vi "parse message read.vi"(9 "# of messages":i32=6, 10 "Raw Data In":u8[](array[numeric])=array[481600 elements]) -> (2 "Messages out":T1[](array[typedef]) {"AckBytes [8]" format="%.0x"; "Data [8]" format="%.0x"; "ArbIDOrHeader" format="%.0x"; "DescriptionID" format="%.0x"; "NetworkID" format="%.0x"})   [LabVIEW 2009]
uses:
  ctl spymessage.ctl
panel:
  out "subarray":u8[][](array[numeric])
  out "Array":u8[](array[numeric])
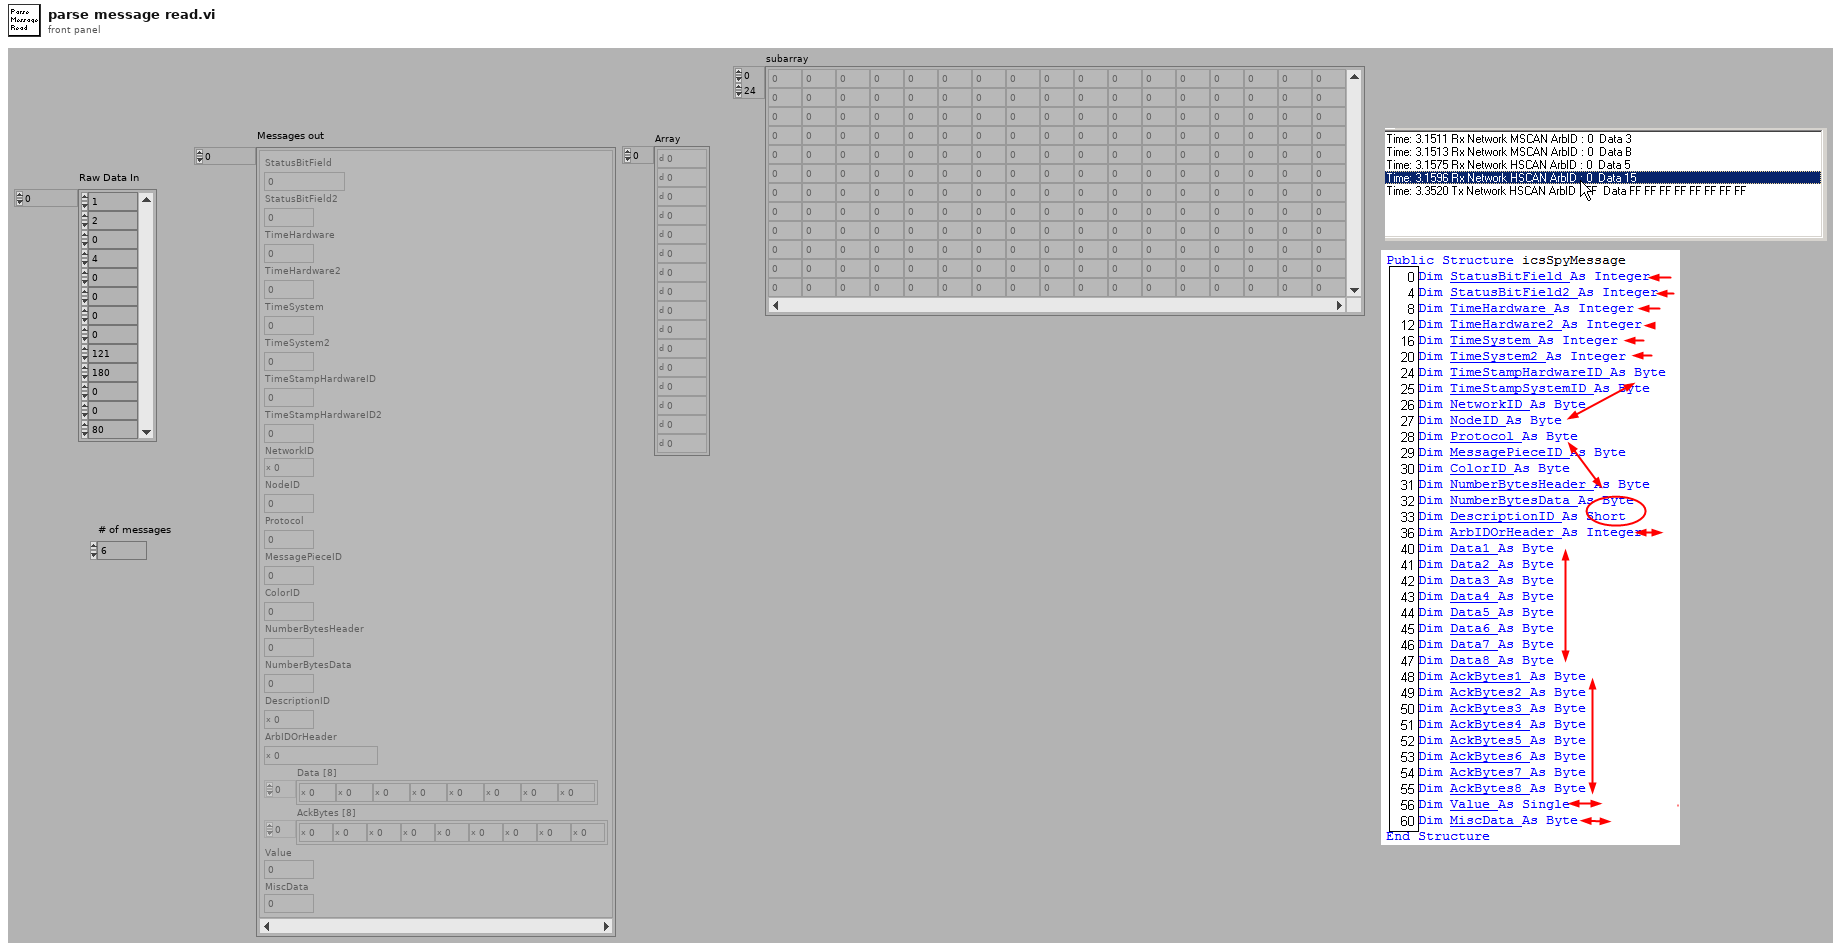
[diagram p1: front panel]
types:
  T1 = typedef "ctl spymessage.ctl" = cluster{"StatusBitField":u32, "StatusBitField2":u32, "TimeHardware":u32, "TimeHardware2":u32, "TimeSystem":u32, "TimeSystem2":u32, "TimeStampHardwareID":u8, "TimeStampHardwareID2":u8, "NetworkID":u8, "NodeID":u8, "Protocol":u8, "MessagePieceID":u8, "ColorID":u8, "NumberBytesHeader":u8, "NumberBytesData":u8, "DescriptionID":u16, "ArbIDOrHeader":u32, "Data [8]":u8[], "AckBytes [8]":u8[], "Value":sgl, "MiscData":u8}
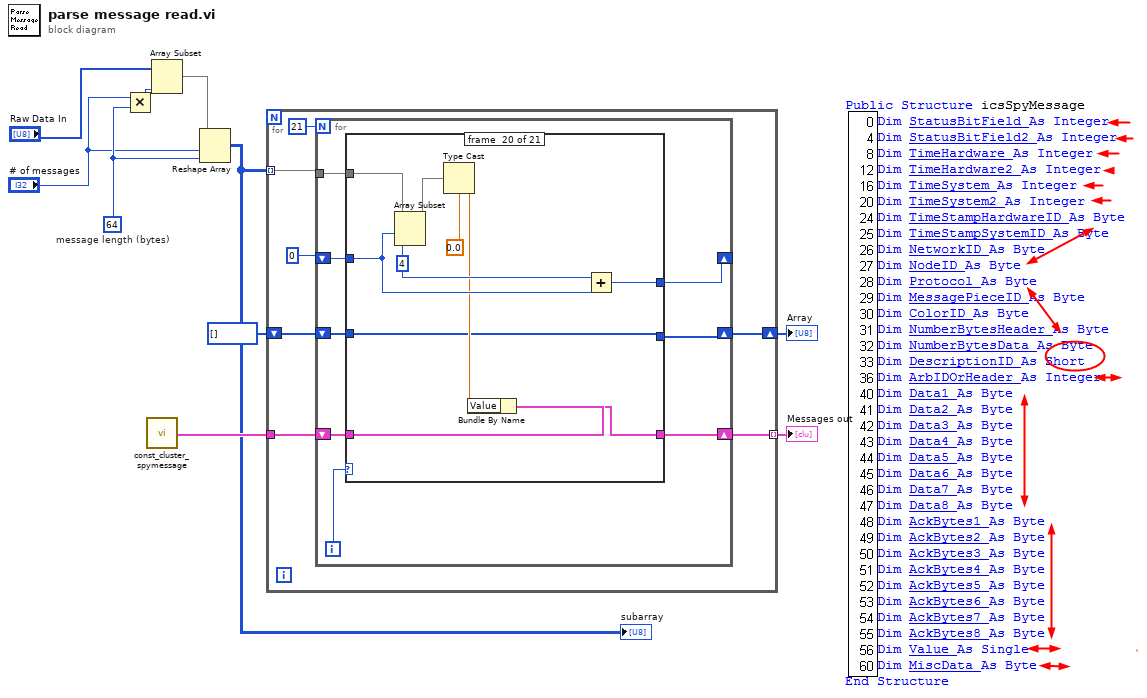
[diagram p0: block diagram]
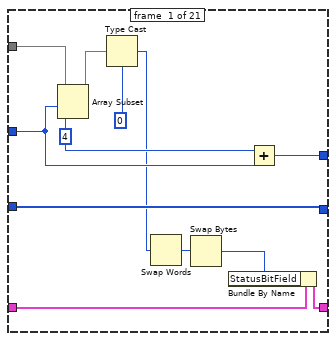
[diagram p2: hidden frame]
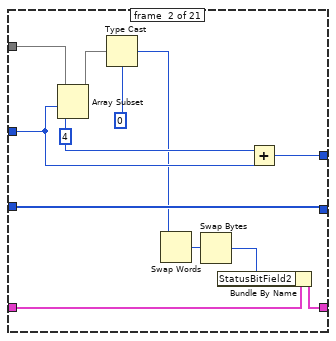
[diagram p3: hidden frame]
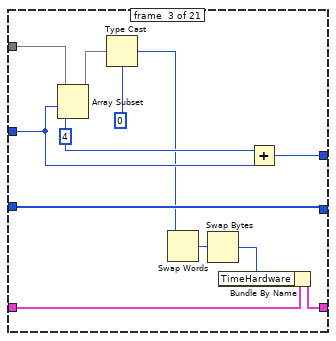
[diagram p4: hidden frame]
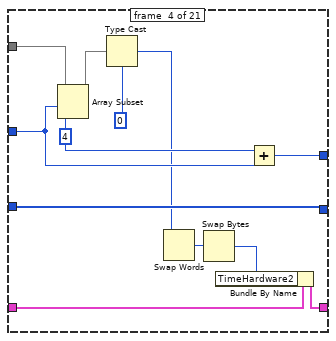
[diagram p5: hidden frame]
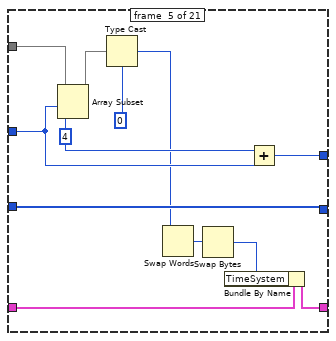
[diagram p6: hidden frame]
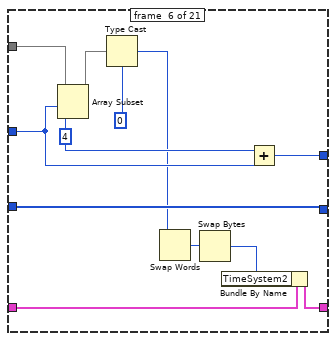
[diagram p7: hidden frame]
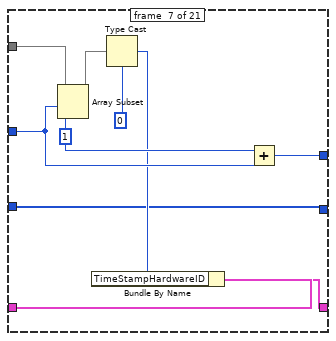
[diagram p8: hidden frame]
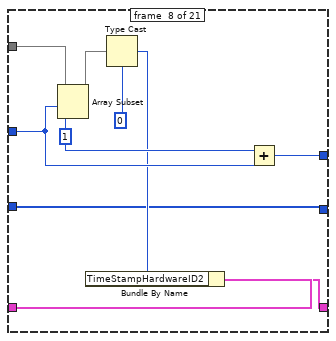
[diagram p9: hidden frame]
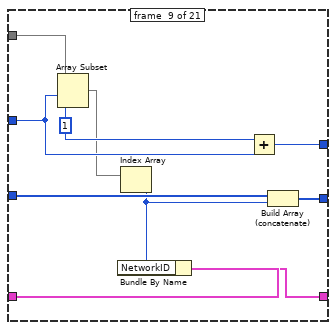
[diagram p10: hidden frame]
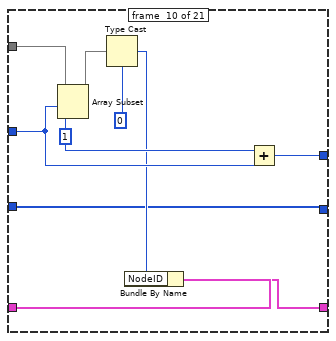
[diagram p11: hidden frame]
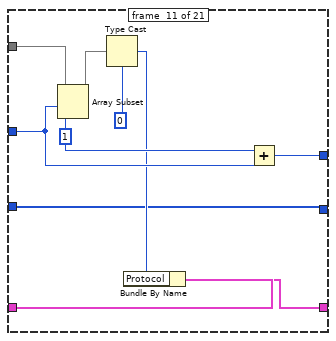
[diagram p12: hidden frame]
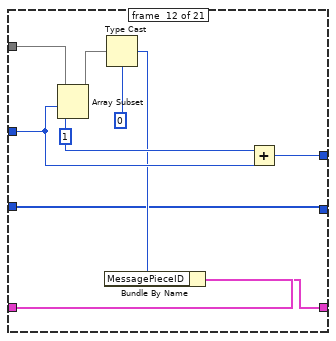
[diagram p13: hidden frame]
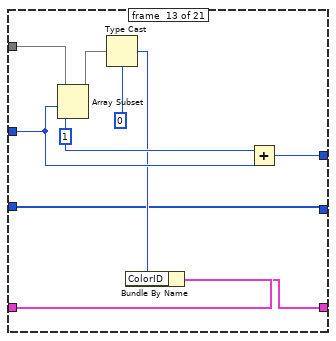
[diagram p14: hidden frame]
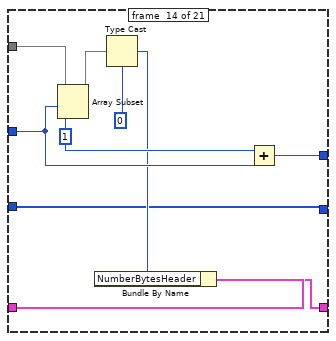
[diagram p15: hidden frame]
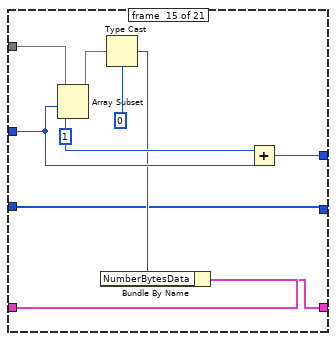
[diagram p16: hidden frame]
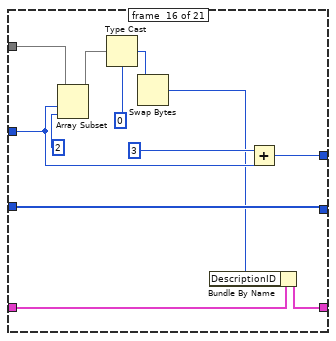
[diagram p17: hidden frame]
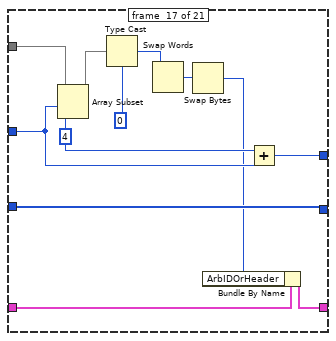
[diagram p18: hidden frame]
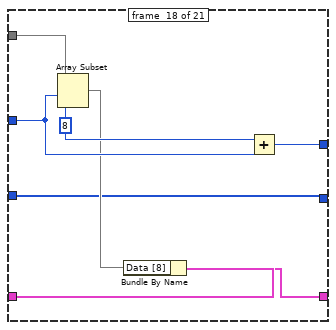
[diagram p19: hidden frame]
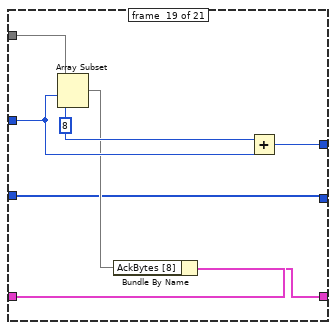
[diagram p20: hidden frame]
diagram:
  w5 = 64  # message length (bytes)
  n1 = Multiply(x="# of messages", y=w5) -> (x*y=w4:i32)
  n2 = call "const_cluster_spymessage.vi"() -> ("SpyMessage{}"=w10:T1)
  n3 = Array Subset(array="Raw Data In", length=w4) -> (w3:u8[])  [unwired: 1 in]
  n4 = Reshape Array(w3, "# of messages", w5) -> (w1:u8[][])
  "subarray" <- w1
  n5 = for {
    tunnel: w1 -> [w17] mode=indexing
    tunnel: w10 -> [w16]
    tunnel: [w13] -> w9 mode=indexing
    shift-right: [w11] -> w7
    shift-left: u8[] [] -> [w12]
    n6 = for {
      N: 21 -> [_]
      tunnel: w17 -> [w25]
      shift-right: [w20] -> _
      shift-left: 0 -> [w21]
      shift-right: [w22] -> w13
      shift-left: w16 -> [w23]
      shift-right: [w18] -> w11
      shift-left: w12 -> [w19]
      i -> [w24]
      n7 = case shown="8" w24 {
        tunnel: w25 -> [w35 w47 w59 w71 w83 w95 w105 w115 w125 w135 w145 w155 w165 w175 w185 w197 w209 w217 w225 w235 w246]
        tunnel: w23 -> [w37 w49 w61 w73 w85 w97 w107 w117 w127 w137 w147 w157 w167 w177 w187 w199 w211 w219 w227 w237 w248]
        tunnel: [w36 w48 w60 w72 w84 w96 w106 w116 w126 w136 w146 w156 w166 w176 w186 w198 w210 w218 w226 w236 w247] -> w22
        tunnel: w21 -> [w34 w46 w58 w70 w82 w94 w104 w114 w124 w134 w144 w154 w164 w174 w184 w196 w208 w216 w224 w234 w245]
        tunnel: [w32 w44 w56 w68 w80 w92 w102 w112 w122 w132 w142 w152 w162 w172 w182 w195 w206 w214 w222 w232 w243] -> w20
        tunnel: w19 -> [w29 w41 w53 w65 w77 w89 w98 w108 w121 w128 w138 w148 w158 w168 w178 w190 w203 w212 w220 w228 w238]
        tunnel: [w29 w41 w53 w65 w77 w89 w98 w108 w120 w128 w138 w148 w158 w168 w178 w190 w203 w212 w220 w228 w238] -> w18
        frame #0 {
          w33 = 4 ("length")
          n8 = Array Subset(array=w35, index=w34, length=w33) -> (w31:u8[])
          n9 = Type Cast(type=u32 0 ("length"), x=w31) -> (*(type *) &x=w27:u32)
          n10 = Swap Words(1:w27) -> (0:w28:u32)
          n11 = Swap Bytes(anything=w28) -> (byte swapped=w26:u32)
          n12 = Bundle By Name(cluster=w37, "StatusBitField"=w26) -> (w36:T1)
          n13 = Add(x=w33, y=w34) -> (x+y=w32:i32)
        }
        frame #1 {
          w45 = 4 ("length")
          n14 = Array Subset(array=w47, index=w46, length=w45) -> (w43:u8[])
          n15 = Type Cast(type=u32 0 ("length"), x=w43) -> (*(type *) &x=w39:u32)
          n16 = Swap Words(1:w39) -> (0:w40:u32)
          n17 = Swap Bytes(anything=w40) -> (byte swapped=w38:u32)
          n18 = Bundle By Name(cluster=w49, "StatusBitField2"=w38) -> (w48:T1)
          n19 = Add(x=w45, y=w46) -> (x+y=w44:i32)
        }
        frame #2 {
          w57 = 4 ("length")
          n20 = Array Subset(array=w59, index=w58, length=w57) -> (w55:u8[])
          n21 = Type Cast(type=u32 0 ("length"), x=w55) -> (*(type *) &x=w51:u32)
          n22 = Swap Words(1:w51) -> (0:w52:u32)
          n23 = Swap Bytes(anything=w52) -> (byte swapped=w50:u32)
          n24 = Bundle By Name(cluster=w61, "TimeHardware"=w50) -> (w60:T1)
          n25 = Add(x=w57, y=w58) -> (x+y=w56:i32)
        }
        frame #3 {
          w69 = 4 ("length")
          n26 = Array Subset(array=w71, index=w70, length=w69) -> (w67:u8[])
          n27 = Type Cast(type=0 ("length"), x=w67) -> (*(type *) &x=w63:i32)
          n28 = Swap Words(1:w63) -> (0:w64:i32)
          n29 = Swap Bytes(anything=w64) -> (byte swapped=w62:i32)
          n30 = Bundle By Name(cluster=w73, "TimeHardware2"=w62) -> (w72:T1)
          n31 = Add(x=w69, y=w70) -> (x+y=w68:i32)
        }
        frame #4 {
          w81 = 4 ("length")
          n32 = Array Subset(array=w83, index=w82, length=w81) -> (w79:u8[])
          n33 = Type Cast(type=0 ("length"), x=w79) -> (*(type *) &x=w75:i32)
          n34 = Swap Words(1:w75) -> (0:w76:i32)
          n35 = Swap Bytes(anything=w76) -> (byte swapped=w74:i32)
          n36 = Bundle By Name(cluster=w85, "TimeSystem"=w74) -> (w84:T1)
          n37 = Add(x=w81, y=w82) -> (x+y=w80:i32)
        }
        frame #5 {
          w93 = 4 ("length")
          n38 = Array Subset(array=w95, index=w94, length=w93) -> (w91:u8[])
          n39 = Type Cast(type=0 ("length"), x=w91) -> (*(type *) &x=w87:i32)
          n40 = Swap Words(1:w87) -> (0:w88:i32)
          n41 = Swap Bytes(anything=w88) -> (byte swapped=w86:i32)
          n42 = Bundle By Name(cluster=w97, "TimeSystem2"=w86) -> (w96:T1)
          n43 = Add(x=w93, y=w94) -> (x+y=w92:i32)
        }
        frame #6 {
          w103 = 1 ("length")
          n44 = Array Subset(array=w105, index=w104, length=w103) -> (w101:u8[])
          n45 = Type Cast(type=u8 0 ("length"), x=w101) -> (*(type *) &x=w99:u8)
          n46 = Bundle By Name(cluster=w107, "TimeStampHardwareID"=w99) -> (w106:T1)
          n47 = Add(x=w103, y=w104) -> (x+y=w102:i32)
        }
        frame #7 {
          w113 = 1 ("length")
          n48 = Array Subset(array=w115, index=w114, length=w113) -> (w111:u8[])
          n49 = Type Cast(type=u8 0 ("length"), x=w111) -> (*(type *) &x=w109:u8)
          n50 = Bundle By Name(cluster=w117, "TimeStampHardwareID2"=w109) -> (w116:T1)
          n51 = Add(x=w113, y=w114) -> (x+y=w112:i32)
        }
        frame #8 {
          w123 = 1 ("length")
          n52 = Array Subset(array=w125, index=w124, length=w123) -> (w119:u8[])
          n53 = Index Array(array=w119) -> (element=w118:u8)  [unwired: 1 in]
          n54 = Bundle By Name(cluster=w127, "NetworkID"=w118) -> (w126:T1)
          n55 = Add(x=w123, y=w124) -> (x+y=w122:i32)
          n56 = Build Array (concatenate)(w121, w118) -> (w120:u8[])
        }
        frame #9 {
          w133 = 1 ("length")
          n57 = Array Subset(array=w135, index=w134, length=w133) -> (w131:u8[])
          n58 = Type Cast(type=u8 0 ("length"), x=w131) -> (*(type *) &x=w129:u8)
          n59 = Bundle By Name(cluster=w137, "NodeID"=w129) -> (w136:T1)
          n60 = Add(x=w133, y=w134) -> (x+y=w132:i32)
        }
        frame #10 {
          w143 = 1 ("length")
          n61 = Array Subset(array=w145, index=w144, length=w143) -> (w141:u8[])
          n62 = Type Cast(type=u8 0 ("length"), x=w141) -> (*(type *) &x=w139:u8)
          n63 = Bundle By Name(cluster=w147, "Protocol"=w139) -> (w146:T1)
          n64 = Add(x=w143, y=w144) -> (x+y=w142:i32)
        }
        frame #11 {
          w153 = 1 ("length")
          n65 = Array Subset(array=w155, index=w154, length=w153) -> (w151:u8[])
          n66 = Type Cast(type=u8 0 ("length"), x=w151) -> (*(type *) &x=w149:u8)
          n67 = Bundle By Name(cluster=w157, "MessagePieceID"=w149) -> (w156:T1)
          n68 = Add(x=w153, y=w154) -> (x+y=w152:i32)
        }
        frame #12 {
          w163 = 1 ("length")
          n69 = Array Subset(array=w165, index=w164, length=w163) -> (w161:u8[])
          n70 = Type Cast(type=u8 0 ("length"), x=w161) -> (*(type *) &x=w159:u8)
          n71 = Bundle By Name(cluster=w167, "ColorID"=w159) -> (w166:T1)
          n72 = Add(x=w163, y=w164) -> (x+y=w162:i32)
        }
        frame #13 {
          w173 = 1 ("length")
          n73 = Array Subset(array=w175, index=w174, length=w173) -> (w171:u8[])
          n74 = Type Cast(type=u8 0 ("length"), x=w171) -> (*(type *) &x=w169:u8)
          n75 = Bundle By Name(cluster=w177, "NumberBytesHeader"=w169) -> (w176:T1)
          n76 = Add(x=w173, y=w174) -> (x+y=w172:i32)
        }
        frame #14 {
          w183 = 1 ("length")
          n77 = Array Subset(array=w185, index=w184, length=w183) -> (w181:u8[])
          n78 = Type Cast(type=u8 0 ("length"), x=w181) -> (*(type *) &x=w179:u8)
          n79 = Bundle By Name(cluster=w187, "NumberBytesData"=w179) -> (w186:T1)
          n80 = Add(x=w183, y=w184) -> (x+y=w182:i32)
        }
        frame #15 {
          n81 = Array Subset(array=w197, index=w196, length=2) -> (w194:u8[])
          n82 = Type Cast(type=u16 0 ("length"), x=w194) -> (*(type *) &x=w189:u16)
          n83 = Swap Bytes(anything=w189) -> (byte swapped=w188:u16)
          n84 = Bundle By Name(cluster=w199, "DescriptionID"=w188) -> (w198:T1)
          n85 = Add(x=3, y=w196) -> (x+y=w195:i32)
        }
        frame #16 {
          w207 = 4 ("length")
          n86 = Array Subset(array=w209, index=w208, length=w207) -> (w205:u8[])
          n87 = Type Cast(type=u32 0 ("length"), x=w205) -> (*(type *) &x=w201:u32)
          n88 = Swap Words(1:w201) -> (0:w202:u32)
          n89 = Swap Bytes(anything=w202) -> (byte swapped=w200:u32)
          n90 = Bundle By Name(cluster=w211, "ArbIDOrHeader"=w200) -> (w210:T1)
          n91 = Add(x=w207, y=w208) -> (x+y=w206:i32)
        }
        frame #17 {
          w215 = 8 ("length")
          n92 = Array Subset(array=w217, index=w216, length=w215) -> (w213:u8[])
          n93 = Bundle By Name(cluster=w219, "Data [8]"=w213) -> (w218:T1)
          n94 = Add(x=w215, y=w216) -> (x+y=w214:i32)
        }
        frame #18 {
          w223 = 8 ("length")
          n95 = Array Subset(array=w225, index=w224, length=w223) -> (w221:u8[])
          n96 = Bundle By Name(cluster=w227, "AckBytes [8]"=w221) -> (w226:T1)
          n97 = Add(x=w223, y=w224) -> (x+y=w222:i32)
        }
        frame #19 {
          w233 = 4 ("length")
          n98 = Array Subset(array=w235, index=w234, length=w233) -> (w230:u8[])
          n99 = Type Cast(type=sgl 0.0 ("length"), x=w230) -> (*(type *) &x=w229:sgl)
          n100 = Bundle By Name(cluster=w237, "Value"=w229) -> (w236:T1)
          n101 = Add(x=w233, y=w234) -> (x+y=w232:i32)
        }
        frame #20 {
          n102 = Array Subset(array=w246, index=w245, length=1) -> (w241:u8[])
          n103 = Type Cast(type=u8 0 ("length"), x=w241) -> (*(type *) &x=w240:u8)
          n104 = Bundle By Name(cluster=w248, "MiscData"=w240) -> (w247:T1)
          n105 = Add(x=4, y=w245) -> (x+y=w243:i32)
        }
      }
    }
  }
  "Messages out" <- w9
  "Array" <- w7
